vi "QTrkComputeLocalizeType.vi"(8 "Clear first four pixels":bool=TRUE, 9 "Normalize profile":bool=TRUE, 10 "2D Localization Type (COM) in":T2, 11 "Z Command (None)":T1) -> (3 "Localize Type + Flags":i32)   [LabVIEW 2011]
uses:
  QTrkLocalizationType.ctl
  QTrkZCommandType.ctl
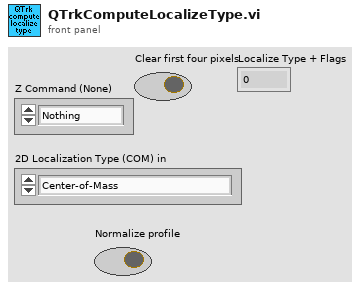
[diagram p1: front panel]
types:
  T1 = typedef "QTrkZCommandType.ctl" = enum16{"Nothing", "ComputeZ"}
  T2 = typedef "QTrkLocalizationType.ctl" = enum16{"Center-of-Mass", "1D Cross-Correlation", "Quadrant Interpolation", "Gaussian 2D MLE", "QI + ZLUTAlign", "ZLUTAlign", "QI + FourierLUT"}
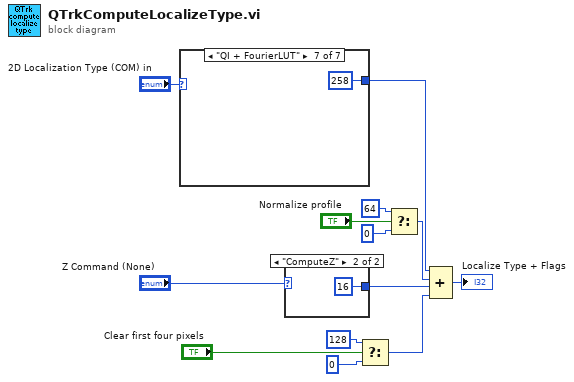
[diagram p0: block diagram]
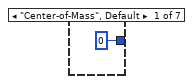
[diagram p2: hidden frame]
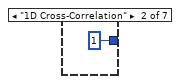
[diagram p3: hidden frame]
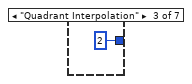
[diagram p4: hidden frame]
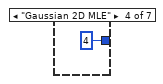
[diagram p5: hidden frame]
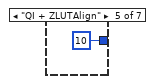
[diagram p6: hidden frame]
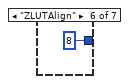
[diagram p7: hidden frame]
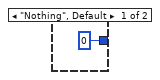
[diagram p8: hidden frame]
diagram:
  n1 = case shown="\"QI + FourierLUT\"" "2D Localization Type (COM) in" {
    tunnel: [0 ("f") 1 ("f") 2 ("f") 4 ("f") 10 ("f") 8 ("f") 258 ("f")] -> w5
    frame "Center-of-Mass", Default {
    }
    frame "1D Cross-Correlation" {
    }
    frame "Quadrant Interpolation" {
    }
    frame "Gaussian 2D MLE" {
    }
    frame "QI + ZLUTAlign" {
    }
    frame "ZLUTAlign" {
    }
    frame "QI + FourierLUT" {
    }
  }
  n2 = case shown="\"ComputeZ\"" "Z Command (None)" {
    tunnel: [0 16] -> w3
    frame "Nothing", Default {
    }
    frame "ComputeZ" {
    }
  }
  n3 = Select(t=128, s="Clear first four pixels", f=0) -> (s? t:f=w2:i32)
  n4 = Select(t=64 ("2D Localization Type (COM) in"), s="Normalize profile", f=0) -> (s? t:f=w4:i32)
  n5 = Compound Arithmetic op=ADD(w5, w4, w3, w2) -> (→"Localize Type + Flags":i32)
